vi "Lock-In Simulator.vi"() -> ()   [LabVIEW 2023]
uses:
  <vilib>/express/express analysis/Spectral/XNode/ExpressSpectralMeasurementsBlockNode.xnode
  <userlib>/_OpenG.lib/appcontrol/appcontrol.llb/openg_application_control.lvlib
  <vilib>/express/express analysis/Spectral/Block/exnSpectralBlock spectral measurements power poly.vi
  <vilib>/express/express analysis/Spectral/Block/exnSpectralBlock spectral measurements power WFM.vi
panel:
  out "XY output":dbl[][](graph)
  out "Lock-in Output":cluster{"Ch 1 Output":dbl, "Ch 2 Output":dbl}(graph)={"Ch 1 Output"=2.99999147666684, "Ch 2 Output"=4.749187889468861e-12} caption="Lock-in Analysis"
  in  "Phase (°)":dbl caption="LOCK-IN Phase" format="%.2f"
  in  "Monitor":u16(ring) items=["Input Signal", "After Mixer"]
  out "Power Spectral Density":cluster{"f0":dbl, "df":dbl, "magnitude":dbl[]}(graph)={"f0"=0.0, "df"=0.01, "magnitude"=[-235.21607825145085, -218.3937535918811, -211.57980464454627, -219.0173516225138, -216.7688290117615, -227.34685181005236, -218.16724192412624, -214.6758364793697, -214.71830862190149, 9.542425094407328, -217.7051009330383, -220.7691633252297, -212.60929639110955, -213.01249803295275, -216.67836056343054, -214.9995950002794, -220.6607411225575, -212.65395812587005, -224.25144059753904, -218.23736966151543, -219.96657196923883, -222.76781056167866, -212.8404028730375, -214.7157786100669, -210.0824382535258, -215.8244598071573, -209.1926052730962, -211.51409381734052, -221.9697489273974, -215.1870579937338, -211.0080371535637, -230.61801872432034, -222.61555635556283, -215.12031239654422, -226.3222143787744, -213.08361230290757, -213.73344693439827, -212.09149744828164, -237.98927548601935, -221.72257852706096, -216.38992841637275, -214.7673342129894, -215.80884880067177, -207.499972356578, -215.86127934217419, -219.33399937224, -219.58911586802202, -216.03742266424695, -215.02006922582063, -218.03690366453156]}
  out "Phasor Representation of Lock-In Output":cluster{"Ch 1 Output":dbl, "Ch 2 Output":dbl}[](graph)=[{"Ch 1 Output"=2.99662702723827, "Ch 2 Output"=-2.5790815749905384e-12}, {"Ch 1 Output"=2.995358935904702, "Ch 2 Output"=-1.600659266616595e-12}, {"Ch 1 Output"=2.9945927518921893, "Ch 2 Output"=-1.1586173268220065e-12}, {"Ch 1 Output"=2.994229007813994, "Ch 2 Output"=-1.0891180515438528e-12}, {"Ch 1 Output"=2.994178400041988, "Ch 2 Output"=-7.018571078375837e-13}, {"Ch 1 Output"=2.9943625860211864, "Ch 2 Output"=1.2387460212332801e-13}, {"Ch 1 Output"=2.9947143595459833, "Ch 2 Output"=9.988247092988941e-13}, {"Ch 1 Output"=2.9951773567757507, "Ch 2 Output"=1.6429471635901913e-12}, {"Ch 1 Output"=2.9957054244850045, "Ch 2 Output"=2.3074000163604176e-12}, {"Ch 1 Output"=2.9962617612040914, "Ch 2 Output"=3.132801941572091e-12}, {"Ch 1 Output"=2.9968179221936446, "Ch 2 Output"=3.8173071586339545e-12}, {"Ch 1 Output"=2.9973527610714332, "Ch 2 Output"=3.922307228194296e-12}, {"Ch 1 Output"=2.9978513646575764, "Ch 2 Output"=3.2926514915426665e-12}, {"Ch 1 Output"=2.998304023363372, "Ch 2 Output"=2.5213873287780478e-12}, {"Ch 1 Output"=2.9987052672430683, "Ch 2 Output"=2.095662338336086e-12}, {"Ch 1 Output"=2.9990529876049297, "Ch 2 Output"=1.7451639948826307e-12}, {"Ch 1 Output"=2.9993476557183225, "Ch 2 Output"=1.0766983637301205e-12}, {"Ch 1 Output"=2.9995916434977667, "Ch 2 Output"=-7.7713426602266e-14}, {"Ch 1 Output"=2.9997886459053773, "Ch 2 Output"=-1.4843901385551484e-12}, {"Ch 1 Output"=2.9999432010043945, "Ch 2 Output"=-2.805711784224486e-12}, {"Ch 1 Output"=3.000060300921067, "Ch 2 Output"=-4.182689754747923e-12}, {"Ch 1 Output"=3.0001450852334033, "Ch 2 Output"=-5.7840254493691e-12}, {"Ch 1 Output"=3.000202607338317, "Ch 2 Output"=-7.433486148990116e-12}, {"Ch 1 Output"=3.0002376639933472, "Ch 2 Output"=-8.674989772490261e-12}, {"Ch 1 Output"=3.000254678334139, "Ch 2 Output"=-9.056488928793801e-12}, {"Ch 1 Output"=3.000257627115586, "Ch 2 Output"=-8.692276282347365e-12}, {"Ch 1 Output"=3.000250003613007, "Ch 2 Output"=-8.104261962935539e-12}, {"Ch 1 Output"=3.0002348084548918, "Ch 2 Output"=-7.494134437440875e-12}, {"Ch 1 Output"=3.0002145615773665, "Ch 2 Output"=-6.9560421124757496e-12}, {"Ch 1 Output"=3.00019132943091, "Ch 2 Output"=-6.736480378543125e-12}, {"Ch 1 Output"=3.0001667624899815, "Ch 2 Output"=-6.884063964721238e-12}, {"Ch 1 Output"=3.000142138997351, "Ch 2 Output"=-7.347238916487514e-12}, {"Ch 1 Output"=3.000118411679514, "Ch 2 Output"=-8.014782704962025e-12}, {"Ch 1 Output"=3.0000962548898635, "Ch 2 Output"=-8.601127070451612e-12}, {"Ch 1 Output"=3.0000761102732425, "Ch 2 Output"=-8.847007531240794e-12}, {"Ch 1 Output"=3.000058229590788, "Ch 2 Output"=-8.936320334688542e-12}, {"Ch 1 Output"=3.000042713802999, "Ch 2 Output"=-8.927590533950898e-12}, {"Ch 1 Output"=3.000029547880391, "Ch 2 Output"=-8.239303128363778e-12}, {"Ch 1 Output"=3.0000186311090906, "Ch 2 Output"=-6.696268700027832e-12}, {"Ch 1 Output"=3.0000098028931537, "Ch 2 Output"=-4.771497592300238e-12}, {"Ch 1 Output"=3.0000028642245966, "Ch 2 Output"=-2.808072656482772e-12}, {"Ch 1 Output"=2.9999975951124305, "Ch 2 Output"=-8.15920048923648e-13}, {"Ch 1 Output"=2.9999937683435385, "Ch 2 Output"=1.160281416825983e-12}, {"Ch 1 Output"=2.9999911599920828, "Ch 2 Output"=2.5866747361203684e-12}, {"Ch 1 Output"=2.9999895571091137, "Ch 2 Output"=3.0453247859602903e-12}, {"Ch 1 Output"=2.999988763022408, "Ch 2 Output"=2.99657373707623e-12}, {"Ch 1 Output"=2.999988600658461, "Ch 2 Output"=3.25905893169565e-12}, {"Ch 1 Output"=2.999988914265522, "Ch 2 Output"=4.051312205799775e-12}, {"Ch 1 Output"=2.999989569881677, "Ch 2 Output"=4.7268767433370936e-12}, {"Ch 1 Output"=2.9999904548535827, "Ch 2 Output"=4.886296431704625e-12}] caption="XY Graph"
  out "Time-Domain":dbl[][](graph)
  in  "Tab Control":enum32{"Main Settings ", "Other Settings"}(tab)
  in  "Sinusoidal Input":cluster{"fc (Hz)":dbl, "Ac (V)":dbl}[](array[cluster])
  in  "Frequency fS (Hz)":dbl=90.0 caption="Frequency" format="%.2f"
  in  "Amplitude AS (V)":dbl=3.0 caption="Amplitude" format="%.2f"
  in  "AM Percentage (%)":dbl caption="Noise Amplitude" min=0.0 max=100.0
  in  "Phase  f (°)":dbl caption="Phase Angle" format="%.2f"
  in  "AM Freq fAM (Hz)":dbl=1.0 caption="Noise Amplitude" format="%.4f"
  in  "Auto-Track":bool=TRUE caption="Auto-Tracking"
  in  "Low-Pass Filter":bool=TRUE
  in  "Time Constant t (s)":dbl=3.0 caption="Time Constant (sec)" format="%#.1p"
  in  "Rolloff":sgl(ring)=2.0 caption="Low-pass filter slope" items=["None", "6 dB/oct", "12 dB/oct", "18 dB/oct", "24 dB/oct"]
  in  "Ref  Freq  fR (Hz)":dbl=90.0 caption="Manual Set" format="%.2f"
  in  "noise (V)":dbl=1e-11 caption="Noise Amplitude" min=1e-11 format="%.4f"
  in  "Enable sinusoidal inputs":bool
  out "CH Y Output (V) 2":dbl format="%#_3p"
  out "CH Y Output (V)":dbl(knob)=2.99999147666684 caption="CH 1 Output" scale=-5.0..5.0
  out "CH X Output (V) 2":dbl format="%#_3p"
  out "CH X Output (V)":dbl(knob)=2.99999147666684 caption="CH 1 Output" scale=-5.0..5.0
  out "Ch 1 Output":dbl=2.99999147666684 format="%.2f"
  out "Ch 2 Output":dbl=4.749187889468861e-12 format="%.2f"
  out "Magnitude":dbl=2.99999147666684 caption="Input Signal Amp" format="%.2f"
  out "Phase":dbl=9.070306509121702e-11 caption="Phase Difference" format="%.2f"
  out "Sampling Freq.":dbl=1000.0 format="%.2f"
  in  "IntegrationPeriod(s)":dbl=0.1 format="%#_6p"
  in  "Sampling Int. (s)":dbl=0.001 caption="Sampling Int. (ms)" format="%.3f"
  # ","
  # "Input Signal"
  # "Lockin Output"
  # "Lockin Settings"
  # "Additional Signals"
  # "Lock-In Output"
  # "Sampling"
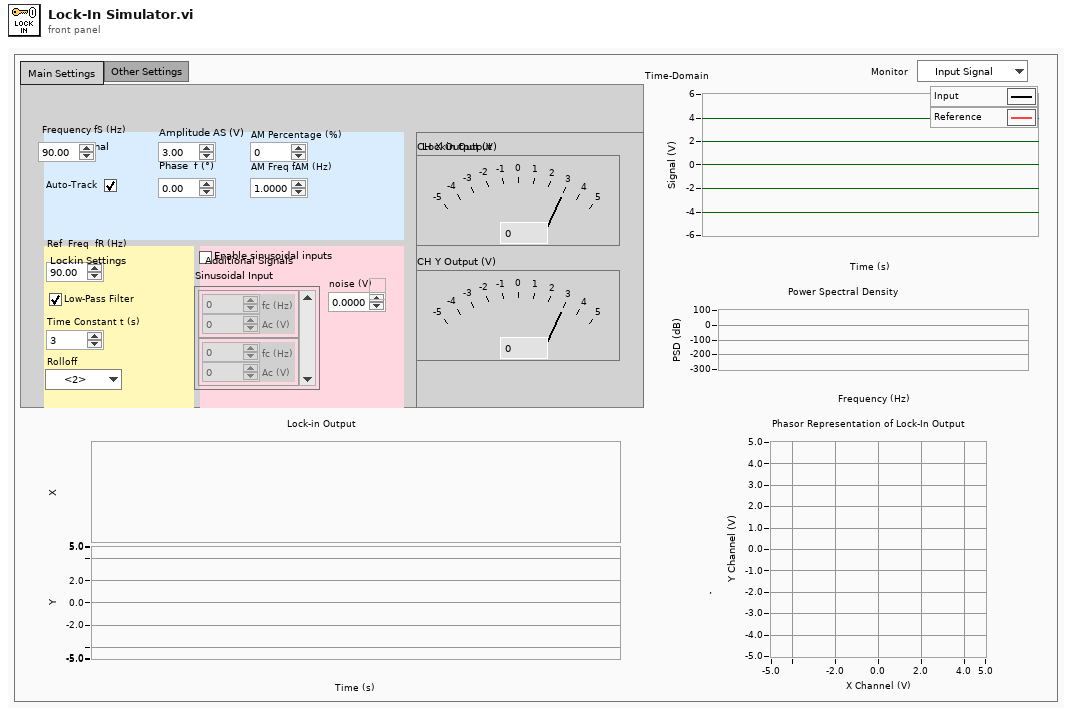
[diagram p1: front panel]
types:
  T1 = cluster{"averaging mode":u16, "weighting mode":u16, "number of averages":u32}
  T2 = cluster{"dB On (F)":bool, "unwrap phase (F)":bool, "convert to degree (F)":bool}
  T3 = cluster{"Amplitude AS (V)":dbl, " Frequency fS (Hz)":dbl, "Phase  f (°)":dbl, dbl, "Rolloff":sgl, "Time Constant t (s)":dbl, bool, " Phase (°)":dbl, " Frequency fS (Hz)":dbl, dbl, "AM Freq fAM (Hz)":dbl, "Sampling Int. (s)":dbl, dbl}
  T4 = cluster{"Amplitude":dbl, "Frequency":dbl, "Phase Angle":dbl, "Spectral Amplitude":dbl, "Time":dbl, "Low-pass filter scope":dbl, "Time Constant (sec)":dbl, "Reset Filters":bool, "LOCK-IN Phase":dbl, "LOCK-IN Freq":dbl, "Sampling-Int(ms)":dbl, "Reference Signal":cluster{dbl[], dbl[]}, "Input Signal":dbl[], "N":i32}
  T5 = cluster{"Amplitude":dbl, "Frequency":dbl, "Phase Angle":dbl, "Noise Amplitude":dbl, "Time":dbl, "Low-pass filter slope":dbl, "Time Constant (sec)":dbl, "Reset Filters":bool, "LOCK-IN Phase":dbl, "LOCK-IN Freq":dbl, "Input Signal":dbl[], "Ch 1 Mult":dbl, "Ch 2 Mult":dbl, "Reference Signal":cluster{dbl[], dbl[]}}
  T6 = cluster{"Ch 1 Output":dbl, "Ch 2 Output":dbl, "Input Signal Amp":dbl, "Phase Difference":dbl, "X-Y Data":cluster{"Current Queue":dbl[], "Current Queue":dbl[]}, "Input Signal":dbl[], "Reference Signal":cluster{dbl[], dbl[]}}
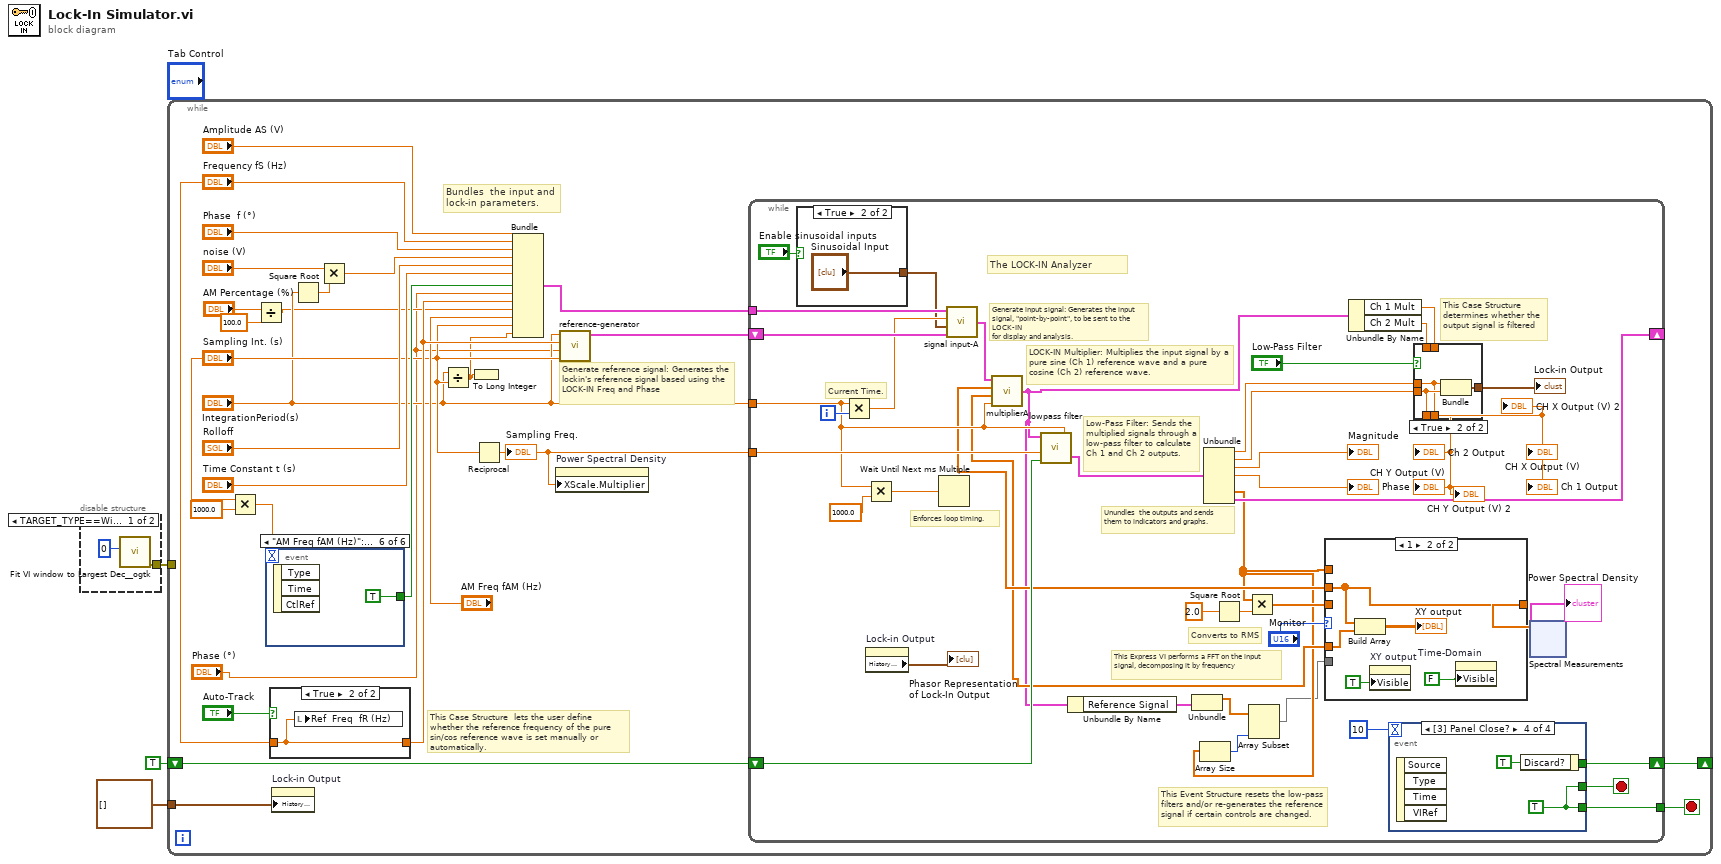
[diagram p0: block diagram]
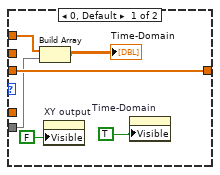
[diagram p3: hidden frame]
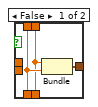
[diagram p4: hidden frame]
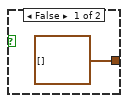
[diagram p5: hidden frame]
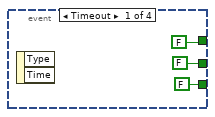
[diagram p6: hidden frame]
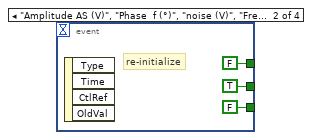
[diagram p7: hidden frame]
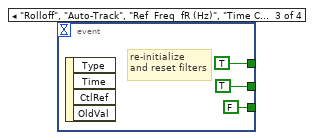
[diagram p8: hidden frame]
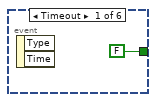
[diagram p9: hidden frame]
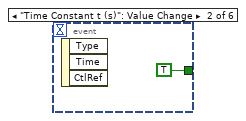
[diagram p10: hidden frame]
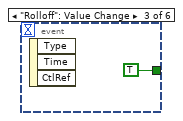
[diagram p11: hidden frame]
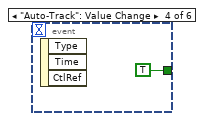
[diagram p12: hidden frame]
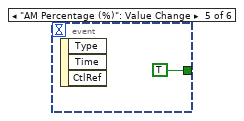
[diagram p13: hidden frame]
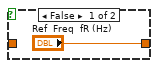
[diagram p14: hidden frame]
diagram:
  n1 = disable-structure shown="TARGET_TYPE==Windows, Default" {
    disable-tunnel: [w5 _] -> w1
    frame condition #0 (active) {
      n2 = call <userlib>:"Fit VI window to Largest Dec__ogtk.vi"("border spacing (2 px)"=0) -> ("error out"=w5:errorcluster)  [unwired: 5 in, 1 out]
    }
    frame condition #1 {
    }
  }
  n3 = while {
    shift-right: [w26] -> _
    shift-left: TRUE -> [w27]
    tunnel: cluster{"Ch 1 Output":dbl, "Ch 2 Output":dbl}[] [] ("History Data") -> [w8]
    tunnel: w1 -> [_]
    stop <- w6 stop-if-true
    # "Generate reference signal: Generates the \nlockin's reference signal based using the \nLOCK-IN Freq and Phase"
    # "This Case Structure  lets the user define whether the reference frequency of the pure sin/cos reference wave is set manually or automatically."
    # "Bundles  the input and lock-in parameters."
    n4 = Multiply(x="Sampling Int. (s)", y=1000.0) -> (x*y=w20:dbl)
    n5 = Divide(x="AM Percentage (%)", y=100.0) -> (x/y=w10:dbl)
    n6 = event shown="[5] \"AM Freq fAM (Hz)\": Value Change" {
      selector: _ -> [_ _ _ _ _ _]
      dyn-events: _ -> [_ _ _ _ _ _]
      timeout: w20 -> [_ _ _ _ _ _]
      tunnel: [FALSE TRUE TRUE TRUE TRUE TRUE] -> w23
      event Timeout {
        n7 = event-data() -> ()  [unwired: 1 in, 2 out]
      }
      event "Time Constant t (s)": Value Change {
        n8 = event-data() -> ()  [unwired: 1 in, 3 out]
      }
      event "Rolloff": Value Change {
        n9 = event-data() -> ()  [unwired: 1 in, 3 out]
      }
      event "Auto-Track": Value Change {
        n10 = event-data() -> ()  [unwired: 1 in, 3 out]
      }
      event "AM Percentage (%)": Value Change {
        n11 = event-data() -> ()  [unwired: 1 in, 3 out]
      }
      event "AM Freq fAM (Hz)": Value Change {
        n12 = event-data() -> ()  [unwired: 1 in, 3 out]
      }
    }
    n13 = case shown="True" "Auto-Track" {
      tunnel: ["Ref  Freq  fR (Hz)" w123] -> w22
      tunnel: "Frequency fS (Hz)" -> [_ w123]
      frame False {
      }
      frame True {
        n14 = local write "Ref  Freq  fR (Hz)"(w123) -> ()
      }
    }
    n15 = property on="Lock-in Output" class="WFChart (strict)"("History Data"=w8) -> ()  [unwired: 2 in, 2 out]
    n16 = Square Root(x="IntegrationPeriod(s)") -> (sqrt(x)=w14:dbl)
    n17 = Multiply(x="noise (V)", y=w14) -> (x*y=w15:dbl)
    n18 = Divide(x="IntegrationPeriod(s)", y="Sampling Int. (s)") -> (x/y=w7:dbl)
    n19 = To Long Integer(number=w7) -> ()  [unwired: 1 out]
    n20 = Reciprocal(x="Sampling Int. (s)") -> (1/x=w28:dbl)
    "Sampling Freq." <- w28
    n21 = Bundle("Amplitude AS (V)"="Amplitude AS (V)", "Frequency fS (Hz)"="Frequency fS (Hz)", "Phase  f (°)"="Phase  f (°)", w15, "Rolloff"="Rolloff", "Time Constant t (s)"="Time Constant t (s)", w23, "Phase (°)"="Phase (°)", "Frequency fS (Hz)"=w22, w10, "AM Freq fAM (Hz)"="AM Freq fAM (Hz)", "Sampling Int. (s)"="Sampling Int. (s)", w7) -> (w30:T3)  [unwired: 1 in]
    n22 = property on="Power Spectral Density" class="WFGraph (strict)"("XScale.Multiplier"=w28) -> ()  [unwired: 2 in, 2 out]
    n23 = call "reference-generator.vi"("SamplingInt(s)"="Sampling Int. (s)", "LockinPhase"="Phase (°)", "LockinFreq"=w22, "IntegrationPeriod(s)"="IntegrationPeriod(s)") -> ("output cluster"=w29:cluster{dbl[], dbl[]})  [unwired: 7 in]
    n24 = while {
      tunnel: w28 -> [w65]
      tunnel: w30 -> [w71]
      tunnel: "IntegrationPeriod(s)" -> [w53]
      shift-right: [w72] -> _
      shift-left: w29 -> [w70]
      shift-right: [w62] -> w26
      shift-left: w27 -> [w63]
      tunnel: [w36] -> w6
      i -> [w68]
      stop <- w64 stop-if-true
      # "This Case Structure  determines whether the output signal is filtered"
      # "Converts to RMS"
      # "This Express VI performs a FFT on the input signal, decomposing it by frequency"
      # "Enforces loop timing."
      # "Current Time."
      # "This Event Structure resets the low-pass filters and/or re-generates the reference signal if certain controls are changed."
      # "The LOCK-IN Analyzer"
      # "Unundles  the outputs and sends them to indicators and graphs."
      # "Low-Pass Filter: Sends the multiplied signals through a low-pass filter to calculate Ch 1 and Ch 2 outputs."
      # "LOCK-IN Multiplier: Multiplies the input signal by a pure sine (Ch 1) reference wave and a pure cosine (Ch 2) reference wave."
      # "Generate input signal: Generates the input signal, \"point-by-point\", to be sent to the LOCK-IN \nfor display and analysis."
      n25 = case shown="True" "Enable sinusoidal inputs" {
        tunnel: [cluster{"F":dbl, "Ampl":dbl}[] [] ("Coherent Noise") "Sinusoidal Input"] -> w55
        frame False {
        }
        frame True {
        }
      }
      n26 = Multiply(x=w53, y=w68) -> (x*y=w69:dbl)
      n27 = Multiply(x=w53, y=1000.0) -> (x*y=w60:dbl)
      n28 = property on="Lock-in Output" class="WFChart (strict)"() -> ("History Data"=→"Phasor Representation of Lock-In Output":cluster{"Ch 1 Output":dbl, "Ch 2 Output":dbl}[])  [unwired: 2 in, 2 out]
      n29 = Wait Until Next ms Multiple(millisecond multiple=w60) -> ()  [unwired: 1 out]
      n30 = call "signal input-A.vi"("Reference Signal"=w70, "Coherent Noise"=w55, "Time"=w69, "Input"=w71) -> ("OUTPUT"=w44:T4)
      n31 = call "multiplierA.vi"("Integration Period (s)"=w53, "Input"=w44) -> ("OUTPUT"=w37:T5, "ymod"=w46:dbl[], "xmod"=w47:dbl[])
      n32 = call "lowpass filter.vi"("Integration Period (s)"=w53, "initialize filters"=w63, "Sampling Freq"=w65, "INPUT"=w37) -> ("OUTPUT"=w66:T6)  [unwired: 1 in]
      n33 = Unbundle By Name(w37) -> ("Reference Signal"=w43:cluster{dbl[], dbl[]})
      n34 = Unbundle(w43) -> (w41:dbl[])  [unwired: 1 out]
      n35 = Unbundle(w66) -> ("Ch 1 Output"=w74:dbl, "Ch 2 Output"=w73:dbl, "Input Signal Amp"=→"Magnitude":dbl, "Phase Difference"=→"Phase":dbl, "Input Signal"=w40:dbl[], "Reference Signal"=w72:cluster{dbl[], dbl[]})  [unwired: 1 out]
      n36 = Array Size(array=w40) -> (size(s)=w42:i32)
      n37 = Square Root(x=2.0) -> (sqrt(x)=w59:dbl)
      n38 = Multiply(x=w40, y=w59) -> (x*y=w50:dbl[])
      n39 = Array Subset(array=w41, length=w42) -> (w39:dbl[])  [unwired: 1 in]
      n40 = case shown="1" "Monitor" {
        tunnel: w50 -> [w82 _]
        tunnel: [w82 w87] -> w49
        tunnel: w47 -> [_ w87]
        tunnel: w40 -> [w81 _]
        tunnel: w46 -> [_ w86]
        tunnel: w39 -> [w80 _]
        frame 0, Default {
          n41 = Build Array(w81, w80) -> (→"Time-Domain":dbl[][])
          n42 = property on="XY output" class="WFGraph (strict)"("Visible"=FALSE) -> ()  [unwired: 2 in, 2 out]
          n43 = property on="Time-Domain" class="WFGraph (strict)"("Visible"=TRUE) -> ()  [unwired: 2 in, 2 out]
        }
        frame 1 {
          n44 = Build Array(w87, w86) -> (→"XY output":dbl[][])
          n45 = property on="XY output" class="WFGraph (strict)"("Visible"=TRUE) -> ()  [unwired: 2 in, 2 out]
          n46 = property on="Time-Domain" class="WFGraph (strict)"("Visible"=FALSE) -> ()  [unwired: 2 in, 2 out]
        }
      }
      n47 = Unbundle By Name(w37) -> ("Ch 1 Mult"=w51:dbl, "Ch 2 Mult"=w52:dbl)
      n48 = event shown="[3] Panel Close?" {
        selector: _ -> [_ _ _ _]
        dyn-events: _ -> [_ _ _ _]
        timeout: 10 -> [_ _ _ _]
        tunnel: [FALSE TRUE TRUE w114] -> w64
        tunnel: [FALSE FALSE TRUE _] -> w62
        tunnel: [FALSE FALSE FALSE w114] -> w36
        event Timeout {
          n49 = event-data() -> ()  [unwired: 1 in, 2 out]
        }
        event "Amplitude AS (V)", "Phase  f (°)", "noise (V)", "Frequency fS (Hz)": Value Change {
          # "re-initialize"
          n50 = event-data() -> ()  [unwired: 1 in, 4 out]
        }
        event "Rolloff", "Auto-Track", "Ref  Freq  fR (Hz)", "Time Constant t (s)", "IntegrationPeriod(s)", "Sampling Int. (s)", "AM Percentage (%)", "AM Freq fAM (Hz)": Value Change {
          # "re-initialize\nand reset filters"
          n51 = event-data() -> ()  [unwired: 1 in, 4 out]
        }
        event Panel Close? {
          w114 = TRUE
          n52 = event-data() -> ()  [unwired: 1 in, 4 out]
          n53 = event-data("Discard?"=TRUE) -> ()  [unwired: 1 in, 1 out]
        }
      }
      n54 = case shown="True" "Low-Pass Filter" {
        tunnel: w74 -> [_ w91]
        tunnel: w73 -> [_ w92]
        tunnel: [w90 w93] -> w45
        tunnel: w52 -> [w89 _]
        tunnel: w51 -> [w88 _]
        tunnel: [w89 w92] -> w34
        tunnel: [w88 w91] -> w35
        frame False {
          n55 = Bundle("Ch 1 Mult"=w88, "Ch 2 Mult"=w89) -> (w90:cluster{"Ch 1 Mult":dbl, "Ch 2 Mult":dbl})  [unwired: 1 in]
        }
        frame True {
          n56 = Bundle("Ch 1 Output"=w91, "Ch 2 Output"=w92) -> (w93:cluster{"Ch 1 Output":dbl, "Ch 2 Output":dbl})  [unwired: 1 in]
        }
      }
      "Ch 1 Output" <- w35
      "Ch 2 Output" <- w34
      "CH X Output (V)" <- w35
      "CH Y Output (V)" <- w34
      "Lock-in Output" <- w45
      "CH X Output (V) 2" <- w35
      "CH Y Output (V) 2" <- w34
      n57 = xnode "Spectral Measurements"("Signals"=w49) -> ("Power Spectrum"=→"Power Spectral Density":cluster{"f0":dbl, "df":dbl, "magnitude":dbl[]})  [unwired: 1 in, 1 out]
    }
  }
